vi "WFM MNGR CLOSE.vi"(8 "error in (no error)":errorcluster, 11 "WFM MNGR in":refnum<class "QPA MSMT Waveform Manager.lvclass">) -> (0 "error out":errorcluster, 3 "WFM MNGR out":refnum<class "QPA MSMT Waveform Manager.lvclass">)   [LabVIEW 2016, in "QPA MSMT Waveform Manager.lvclass"]
uses:
  QPA MSMT Waveform Manager.lvclass
  QPA MSMT Waveform Manager.lvclass/QPA MSMT Waveform Manager.ctl
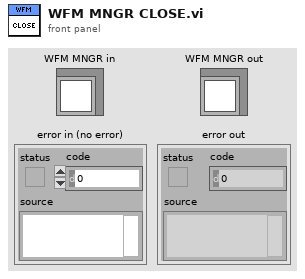
[diagram p1: front panel]
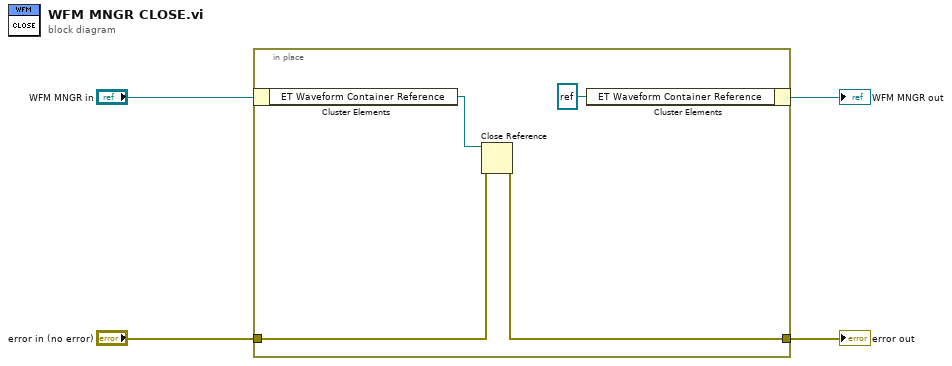
[diagram p0: block diagram]
diagram:
  n1 = in-place {
    in-place-border: "error in (no error)" -> [w6]
    in-place-border: [w5] -> w1
    n2 = in-place-cluster #1("WFM MNGR in") -> ("ET Waveform Container Reference"=w8:refnum<k7>)
    n3 = Close Reference(reference=w8, error in (no error)=w6) -> (error out=w5:errorcluster)
    n4 = in-place-cluster #1("ET Waveform Container Reference"=refnum<k7> refnum) -> (→"WFM MNGR out":refnum<class "QPA MSMT Waveform Manager.lvclass">)
  }
  "error out" <- w1
